vi "CanControlStart.vi"(3 "error in":errorcluster {"code" format="%.0x"}, 4 "start":bool, 5 "CAN Control Handle in":u32 format="%x") -> (0 "error out":errorcluster {"code" format="%.0x"}, 1 "is started":bool, 2 "CAN Control Handle out":u32)   [LabVIEW 2011]
doc: "Starts or stops the CAN controller."
uses:
  vcilva.dll
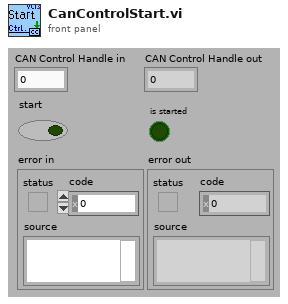
[diagram p1: front panel]
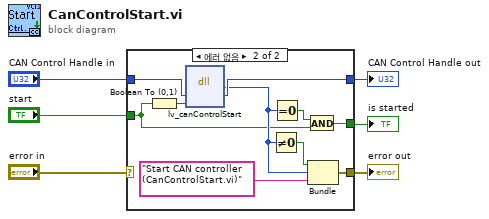
[diagram p0: block diagram]
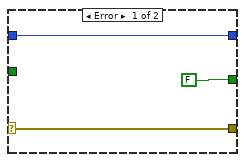
[diagram p2: hidden frame]
diagram:
  n1 = case shown="에러 없음" "error in" {
    selector: "error in" -> [w8 _]
    tunnel: [w8 w19] -> w3
    tunnel: "CAN Control Handle in" -> [w9 w15]
    tunnel: [w9 w14] -> w5
    tunnel: [FALSE w10] -> w2
    tunnel: "start" -> [_ w11]
    frame Error {
    }
    frame No Error {
      n2 = Boolean To (0,1)(Boolean=w11) -> (0, 1=w16:i16)
      n3 = dll-call lib="vcilva.dll" fn="lv_canControlStart"("hCanCtl"=w15, "fStart"=w16) -> (w13:i32, "hCanCtl"=w14:u32)  [unwired: 4 in, 2 out]
      n4 = Not Equal To 0?(x=w13) -> (x != 0?=w18:bool)
      n5 = Equal To 0?(x=w13) -> (x = 0?=w12:bool)
      n6 = And(x=w12, y=w11) -> (x .and. y?=w10:bool)
      n7 = Bundle(w18, w13, "Start CAN controller (CanControlStart.vi)") -> (w19:errorcluster)  [unwired: 1 in]
    }
  }
  "error out" <- w3
  "CAN Control Handle out" <- w5
  "is started" <- w2
